vi "Test.vi"   [LabVIEW 2017]
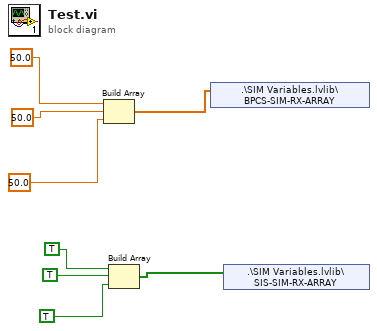
[diagram p0: block diagram]
diagram:
  n1 = Build Array(50.0, 50.0, 50.0) -> (w5:dbl[])
  n2 = Build Array(TRUE, TRUE, TRUE) -> (w1:bool[])
  n3 = shared-variable ".\\SIM Variables.lvlib\\BPCS-SIM-RX-ARRAY"(w5) -> ()  [unwired: 1 in, 1 out]
  n4 = shared-variable ".\\SIM Variables.lvlib\\SIS-SIM-RX-ARRAY"(w1) -> ()  [unwired: 1 in, 1 out]
